vi "Generate Response Paramters.vi"(8 "Error In":errorcluster, 10 "Response String":string, 11 "Response Channel in":T1 format="%.0x") -> (0 "Error Out":errorcluster, 1 "Wait Channel Ref out":T1 format="%.0x", 2 "Linked Channels":T2[](array[typedef]) {"Channel Refnum" format="%.0x"}, 3 "Response Channel out":T1 format="%.0x")   [LabVIEW 2018, in "Instrument Addon Scripting API Messages Unit Tests.lvclass"]
uses:
  Instrument Addon Scripting API Messages Unit Tests.lvclass
  <vilib>/NI Veristand/Custom Device API/Custom Device Item Ref.ctl
  APIs/Scripting API/TypeDefs/Linked Channel.ctl
  <vilib>/NI Veristand/Custom Device API/Custom Device API.lvlib
  APIs/Scripting API/Instrument Addon Scripting API.lvlib
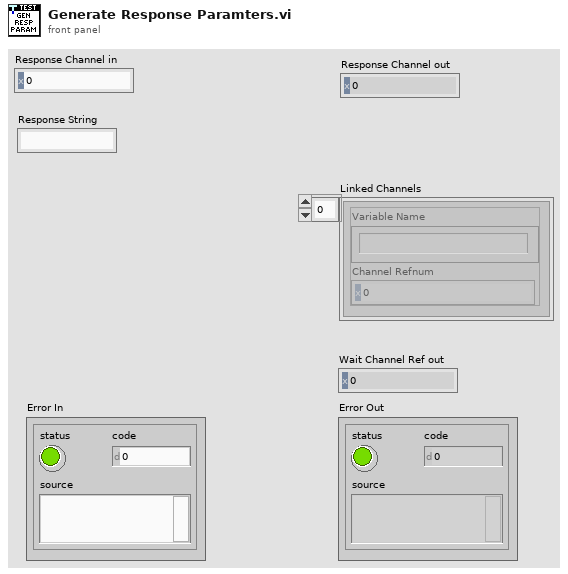
[diagram p1: front panel]
types:
  T1 = typedef "Custom Device API.lvlib/Custom Device Item Ref.ctl" = u64
  T2 = typedef "Instrument Addon Scripting API.lvlib/Linked Channel.ctl" = cluster{"Variable Name":string, "Channel Refnum":T1}
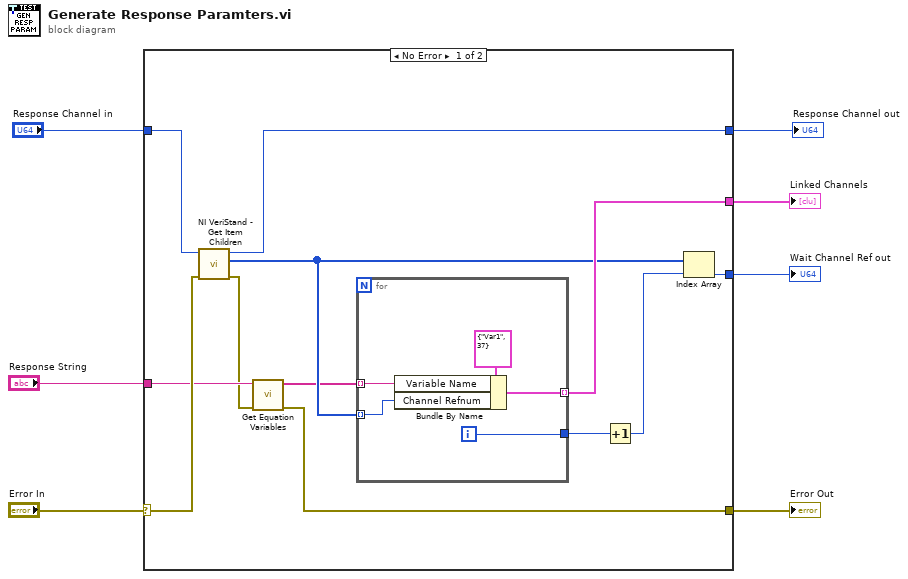
[diagram p0: block diagram]
diagram:
  n1 = case shown="No Error" "Error In" {
    selector: "Error In" -> [w13 w26]
    tunnel: [w19 _] -> w7
    tunnel: [w18 _] -> w6
    tunnel: "Response String" -> [w11 _]
    tunnel: [w8 w26] -> w3
    tunnel: "Response Channel in" -> [w15 w25]
    tunnel: [w12 w25] -> w1
    frame No Error {
      n2 = call <vilib>:"NI VeriStand - Get Item Children.vi"("error in (no error)"=w13, "Item Ref in"=w15) -> ("error out"=w9:errorcluster, "Child Refs"=w14:T1[], "Item Ref out"=w12:T1)  [unwired: 6 in, 1 out]
      n3 = call "Get Equation Variables.vi"("error in (no error)"=w9, "Format String"=w11) -> ("error out"=w8:errorcluster, "Variables out"=w10:string[])  [unwired: 7 in, 1 out]
      n4 = for {
        tunnel: w10 -> [w23] mode=indexing
        tunnel: w14 -> [w22] mode=indexing
        tunnel: [w21] -> w18 mode=indexing
        tunnel: [w20] -> w16
        i -> [w20]
        n5 = Bundle By Name(cluster=T2 {"Variable Name"="Var1", "Channel Refnum"=37} ("Linked Channel"), "Variable Name"=w23, "Channel Refnum"=w22) -> (w21:T2)
      }
      n6 = Increment(x=w16) -> (x+1=w17:i32)
      n7 = Index Array(array=w14, index=w17) -> (element=w19:T1)
    }
    frame Error {
    }
  }
  "Wait Channel Ref out" <- w7
  "Linked Channels" <- w6
  "Error Out" <- w3
  "Response Channel out" <- w1
